vi "Sinusoidal Extraction.vi"() -> ()   [LabVIEW 2014, in "Melody Extraction.lvlib"]
uses:
  Melody Extraction.lvlib
  <vilib>/Math Plots/3D Math Plots/3D Scatter/3D Scatter XCtrl/3D Scatter.xctl
  <vilib>/addons/Sound and Vibration/svt_Weighting/SVT A, B, C Weighting Filter (Fixed Rates) (1 Ch).vi
  <vilib>/Math Plots/3D Math Plots/3D Scatter/3D Scatter Datatype/Public/Plot Helper (Vector).vi
  <vilib>/addons/Sound and Vibration/svt_Weighting/SoundVib_ABCWeighting.lvlib
  <vilib>/Math Plots/3D Math Plots/3D Scatter/3D Scatter Datatype/3D Scatter Datatype.lvclass
panel:
  out "3D Scatter":refnum<class "3D Plot Datatype.lvclass">[](xcontrol)
  in  "Reading Interface":enum32{"Read MP3", "Read generated waveform"}(tab)
  in  "Complete File?":bool
  in  "Seconds to read":dbl
  in  "Input File":path=path "C:/Users/Dany/Documents/GitHub/LabVIEW/Slow-Down_Pitch-Detection/01-23- Summertime.mp3"
  in  "Generated Signal Configuration":T1={"signal type"=enum."Sine Wave", "frequency"=1000.0, "sampling info"={"Sampling Rate"=44100.0, "# Samples"=10000.0}} {"frequency" format="%#_13g"}
  out "Intensity Graph":dbl[][](graph)
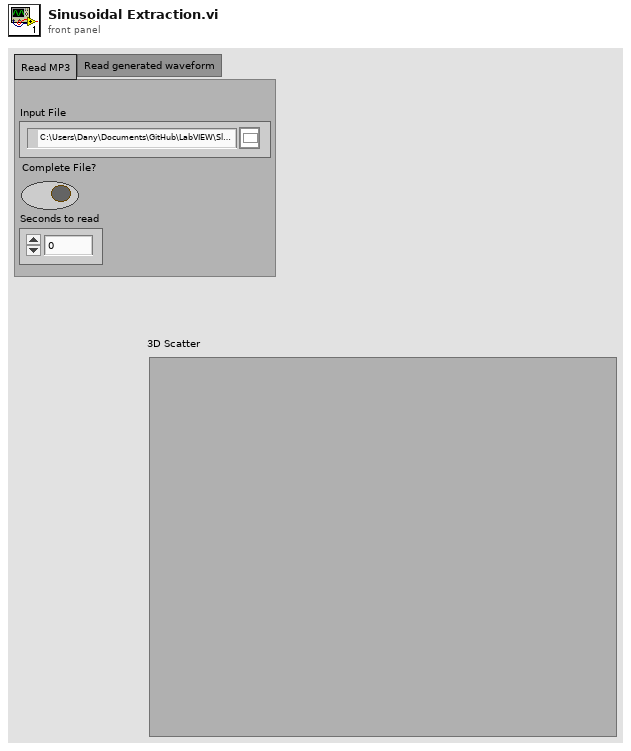
[diagram p1: front panel]
types:
  T1 = cluster{"signal type":enum16{"Sine Wave", "Triangle Wave", "Square Wave", "Sawtooth Wave"}, "frequency":dbl, "sampling info":cluster{"Sampling Rate":dbl, "# Samples":dbl}}
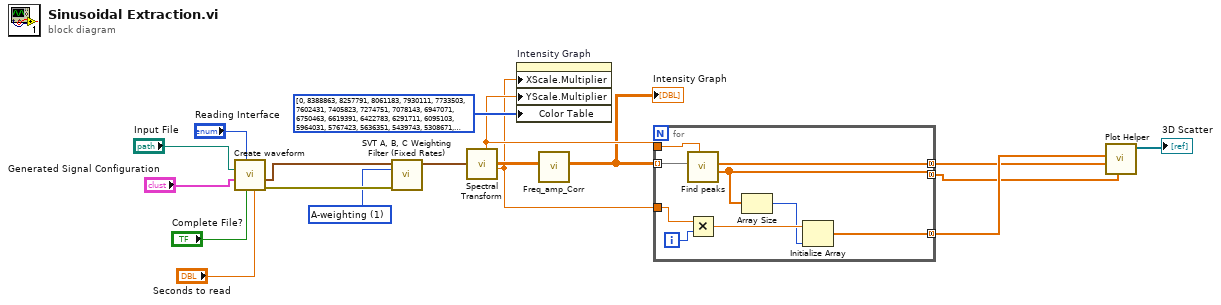
[diagram p0: block diagram]
diagram:
  w15 = u16 1 items=["Linear", "A-weighting", "B-weighting", "C-weighting"] ("weighting")
  n1 = call "Create waveform.vi"("Seconds to read"="Seconds to read", "Complete File?"="Complete File?", "Reading Interface"="Reading Interface", "Generated Signal Configuration"="Generated Signal Configuration", "Input File"="Input File") -> ("error out"=w18:errorcluster, "output waveform"=w9:waveform(dbl))  [unwired: 5 in]
  n2 = call-poly <vilib>:"SVT A, B, C Weighting Filter (Fixed Rates).vi"("error in (no error)"=w18, "weighting"=w15, "scaled signal [EU]"=w9) -> ("weighted signal [EU]"=w17:waveform(dbl))  [unwired: 6 in, 1 out]
  n3 = call "Spectral Transform.vi"("Input Waveform"=w17) -> ("Time Axis Scale Factor"=w5:dbl, "STFT"=w16:dbl[][], "Frequency Axis Scale Factor"=w7:dbl)  [unwired: 8 in]
  n4 = property on="Intensity Graph" class="IntGraph (strict)"("XScale.Multiplier"=w5, "YScale.Multiplier"=w7, "Color Table"=u32[] [0, 8388863, 8257791, 8061183, 7930111, 7733503, 7602431, 7405823, 7274751, 7078143, 6947071, 6750463, 6619391, 6422783, 6291711, 6095103, 5964031, 5767423, 5636351, 5439743, 5308671, 5112063, 4980991, 4784383, 4653311, 4456703, 4325631, 4129023, 3932415, 3801343, 3604735, 3473663, 3277055, 3145983, 2949375, 2818303, 2621695, 2490623, 2294015, 2162943, 1966335, 1835263, 1638655, 1507583, 1310975, 1179903, 983295, 852223, 655615, 524543, 327935, 196863, 511, 1791, 3071, 4351, 5631, 6911, 8191, 9471, 10751, 12031, 13311, 14591, 15871, 17151, 18431, 19711, 20991, 22271, 23551, 24831, 26111, 27391, 28671, 29951, 31231, 32511, 33791, 35071, 36351, 37631, 38911, 40191, 41471, 42751, 44031, 45311, 46591, 47871, 49151, 50431, 51711, 52991, 54271, 55551, 56831, 58111, 59391, 60671, 61951, 63231, 64511, 65532, 65527, 65522, 65517, 65512, 65507, 65502, 65497, 65492, 65487, 65482, 65477, 65472, 65467, 65462, 65457, 65452, 65447, 65442, 65437, 65432, 65427, 65422, 65417, 65412, 65407, 65402, 65397, 65392, 65387, 65382, 65377, 65372, 65367, 65362, 65357, 65352, 65347, 65342, 65337, 65332, 65327, 65322, 65317, 65312, 65307, 65302, 65297, 65292, 65287, 65282, 261888, 589568, 917248, 1244928, 1572608, 1900288, 2227968, 2555648, 2883328, 3211008, 3538688, 3866368, 4194048, 4521728, 4849408, 5177088, 5504768, 5832448, 6160128, 6487808, 6815488, 7143168, 7470848, 7798528, 8126208, 8453888, 8781568, 9109248, 9436928, 9764608, 10092288, 10419968, 10747648, 11075328, 11403008, 11730688, 12058368, 12386048, 12713728, 13041408, 13369088, 13696768, 14024448, 14352128, 14679808, 15007488, 15335168, 15662848, 15990528, 16318208, 16645888, 16775936, 16774656, 16773376, 16772096, 16770816, 16769536, 16768256, 16766976, 16765696, 16764416, 16763136, 16761856, 16760576, 16759296, 16758016, 16756736, 16755456, 16754176, 16752896, 16751616, 16750336, 16749056, 16747776, 16746496, 16745216, 16743936, 16742656, 16741376, 16740096, 16738816, 16737536, 16736256, 16734976, 16733696, 16732416, 16731136, 16729856, 16728576, 16727296, 16726016, 16724736, 16723456, 16722176, 16720896, 16719616, 16718336, 16717056, 16715776, 16714496, 16713216, 16711680] ("rainbow")) -> ()  [unwired: 2 in, 2 out]
  n5 = call "Freq_amp_Corr.vi"("Input STFT"=w16) -> ("Output STFT"=w6:dbl[][])  [unwired: 10 in]
  "Intensity Graph" <- w6
  n6 = for {
    tunnel: w6 -> [w27] mode=indexing
    tunnel: w7 -> [w26]
    tunnel: w5 -> [w25]
    tunnel: [w23] -> w2 mode=concatenating
    tunnel: [w21] -> w1 mode=concatenating
    tunnel: [w19] -> w3 mode=concatenating
    i -> [w24]
    n7 = call "Find peaks.vi"("Frequency Axis Scale Factor"=w26, "FFT (single frame)"=w27) -> ("Peak Magnitudes"=w21:dbl[], "Peaks Frequencies"=w23:dbl[])  [unwired: 8 in]
    n8 = Multiply(x=w25, y=w24) -> (x*y=w22:dbl)
    n9 = Array Size(array=w21) -> (size(s)=w20:i32)
    n10 = Initialize Array(w22, w20) -> (w19:dbl[])
  }
  n11 = call-poly <vilib>:"Plot Helper.vi"("z vector"=w1, "y vector"=w2, "x vector"=w3) -> ("3D Plot lvclass Array out"=→"3D Scatter":refnum<class "3D Plot Datatype.lvclass">[])  [unwired: 3 in, 5 out]
